vi "Create Evaluations.vi"(8 "error in (no error)":errorcluster, 11 "SPECAN_IQSLOT in":refnum<class "SPECAN_IQSLOT.lvclass">) -> (0 "error out":errorcluster, 1 "Evaluations Out":T1[](array[typedef]) {"Low Limit" format="%#_13g"; "SI Scaling" items=["femto"=-15, "pico"=-12, "nano"=-9, "micro"=-6, "milli"=-3, "percent"=-2, ""=0, "kilo"=3, "mega"=6, "giga"=9, "tera"=12]}, 3 "SPECAN_IQSLOT out":refnum<class "SPECAN_IQSLOT.lvclass">)   [LabVIEW 2018, in "SPECAN_IQSLOT.lvlib" / "SPECAN_IQSLOT.lvclass"]
uses:
  SPECAN_IQSLOT.lvclass
  C:/Sequence Automation/Plugins/Measurement Interface.lvlibp/Measurement Interface.lvclass
  Plugins/TestStand API Tools (TSAT).lvlibp/Evaluation Actions/Includes/Controls/TSAT Evaluation.ctl
  Plugins/TestStand API Tools (TSAT).lvlibp/Evaluation Actions/Includes/Controls/TSAT Eval SI Unit Scaling.ctl
  Plugins/TestStand API Tools (TSAT).lvlibp/Evaluation Actions/Includes/Controls/TSAT Evaluation Type.ctl
  Plugins/Measurement Interface.lvlibp/Private Methods/Measurement Name/Read Measurement Name.vi
  Plugins/SeqAuto Evaluations.lvlibp/HiSi/SpecAn_IQSLOT/HiSi_SpecAn_IQSLOT.lvclass
  Plugins/TestStand API Tools (TSAT).lvlibp/Evaluation Actions/TSAT Evaluation Actions.lvlib
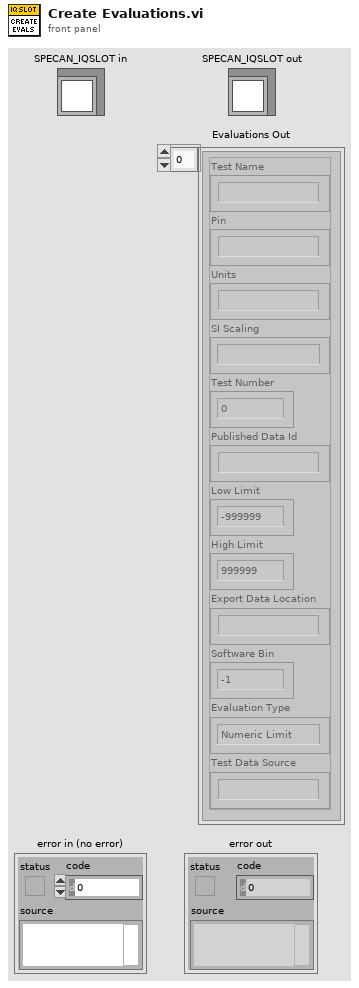
[diagram p1: front panel]
types:
  T1 = typedef "TestStand API Tools (TSAT).lvlibp/TSAT Evaluation Actions.lvlib/TSAT Evaluation.ctl" = cluster{"Test Name":string, "Pin":string, "Units":string, "SI Scaling":T2, "Test Number":i32, "Published Data Id":string, "Low Limit":dbl, "High Limit":dbl, "Export Data Location":string, "Software Bin":i64, "Evaluation Type":T3, "Test Data Source":string}
  T2 = typedef "TestStand API Tools (TSAT).lvlibp/TSAT Evaluation Actions.lvlib/TSAT Eval SI Unit Scaling.ctl" = i16
  T3 = typedef "TestStand API Tools (TSAT).lvlibp/TSAT Evaluation Actions.lvlib/TSAT Evaluation Type.ctl" = enum16{"Numeric Limit", "Pass/Fail", "None"}
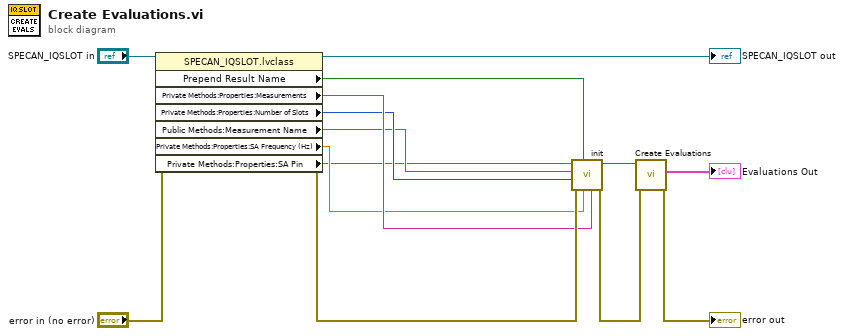
[diagram p0: block diagram]
diagram:
  n1 = property class="SPECAN_IQSLOT.lvclass"(reference="SPECAN_IQSLOT in", error in="error in (no error)") -> (reference out=→"SPECAN_IQSLOT out":refnum<class "SPECAN_IQSLOT.lvclass">, error out=w11:errorcluster, "Prepend Result Name"=w6:bool, "Private Methods:Properties:Measurements"=w5:string, "Private Methods:Properties:Number of Slots"=w4:i32, "Public Methods:Measurement Name"=w2:string, "Private Methods:Properties:SA Frequency (Hz)"=w3:dbl, "Private Methods:Properties:SA Pin"=w1:string)
  n2 = call "init.vi"("Measurements"=w5, "SA Frequency (Hz)"=w3, "Prepend Result Name"=w6, "error in (no error)"=w11, "Number of Slots"=w4, "Measurement Name"=w2, "SA Pin"=w1) -> ("error out"=w9:errorcluster, "Skyworks_PA_Modeswitch_out"=w10:refnum<class "HiSi_SpecAn_IQSLOT.lvclass">)  [unwired: 3 in]
  n3 = call-dynamic "Create Evaluations.vi"("error in (no error)"=w9, "IEvaluation in"=w10) -> ("error out"=→"error out":errorcluster, "Evaluations Out"=→"Evaluations Out":T1[])  [unwired: 7 in, 1 out]
